vi "平行样启动参数选择对话框.vi"() -> (2 "确定启动":bool, 3 "启动模块":T1)   [LabVIEW 2016, in "质控单元.lvlib"]
panel:
  in  "CODCr":bool
  in  "总氮":bool
  in  "确定":bool
  in  "CODMn":bool
  in  "总磷":bool
  in  "取消":bool
  in  "氨氮":bool
  # "请选择平行样测试模块"
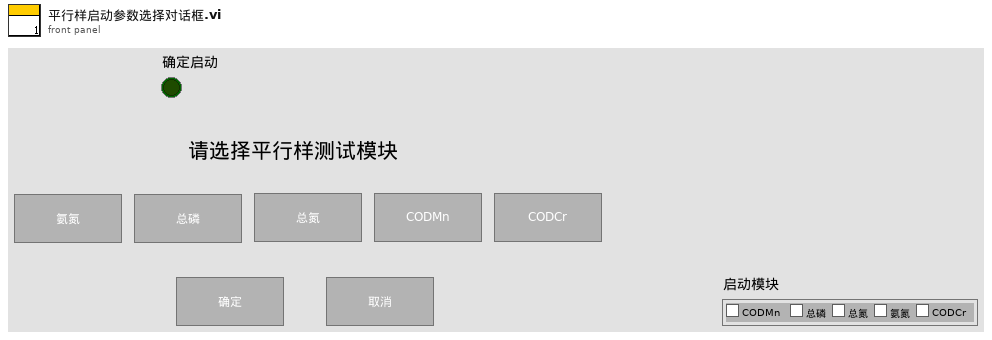
[diagram p1: front panel]
types:
  T1 = cluster{"CODMn":bool, "总磷":bool, "总氮":bool, "氨氮":bool, "CODCr":bool}
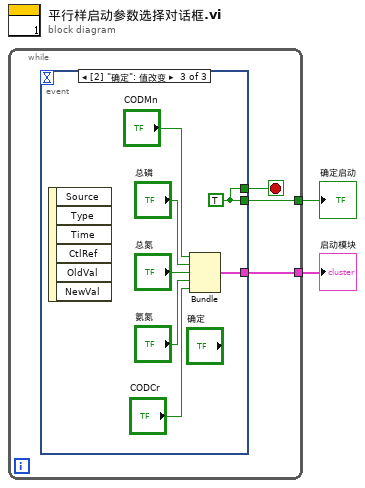
[diagram p0: block diagram]
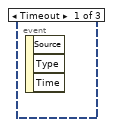
[diagram p2: hidden frame]
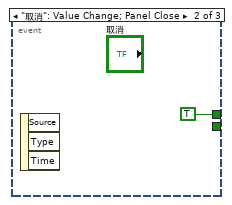
[diagram p3: hidden frame]
diagram:
  n1 = while {
    tunnel: [w4] -> w2
    tunnel: [w3] -> w1
    stop <- w5 stop-if-true
    n2 = event shown="[2] \"确定\": 值改变" {
      selector: _ -> [_ _ _]
      dyn-events: _ -> [_ _ _]
      timeout: _ -> [_ _ _]
      tunnel: [_ TRUE ("确定") w13] -> w5
      tunnel: [_ _ w13] -> w4
      tunnel: [_ _ w9] -> w3
      event Timeout {
        n3 = event-data() -> ()  [unwired: 1 in, 3 out]
      }
      event "取消": Value Change; Panel Close {
        n4 = event-data() -> ()  [unwired: 1 in, 3 out]
      }
      event "确定": Value Change {
        w13 = TRUE ("确定")
        n5 = event-data() -> ()  [unwired: 1 in, 6 out]
        n6 = Bundle("CODMn"="CODMn", "总磷"="总磷", "总氮"="总氮", "氨氮"="氨氮", "CODCr"="CODCr") -> (w9:T1)  [unwired: 1 in]
      }
    }
  }
  "确定启动" <- w2
  "启动模块" <- w1
